vi "Initialize Sink.vi"(11 "Network Sink in":refnum<class "Network Sink.lvclass">) -> (0 "error out":errorcluster, 3 "Network Sink out":refnum<class "Network Sink.lvclass">)   [LabVIEW 2017, in "Network Sink.lvlib" / "Network Sink.lvclass"]
uses:
  <vilib>/gpm_packages/@cs/event-logger/Source/Network Sink/Network Sink/Network Sink.lvclass
  <vilib>/gpm_packages/@cs/event-logger/Source/Network Sink/Network Sink/Network Sink.lvclass/Network Sink.ctl
  <vilib>/gpm_packages/@cs/event-logger/Source/Network Sink/LogEventMessageProtocol/LogEventMessageProtocol.lvclass
  C:/Program Files/National Instruments/LabVIEW 2017/vi.lib/gpm_packages/@cs/Network-sink/Source/Network Interface/IMessagingProtocol/IMessagingProtocol.lvclass
  <vilib>/gpm_packages/@cs/Network-Sink/Source/TCP Interface/TCP Client/TCP Client.lvclass
  C:/Program Files/National Instruments/LabVIEW 2017/vi.lib/gpm_packages/@cs/Network-sink/Source/Network Interface/IConnectionFactory/IConnectionFactory.lvclass
  <vilib>/gpm_packages/@cs/event-logger/Source/Network Sink/SessionHandler/SessionHandler.lvclass
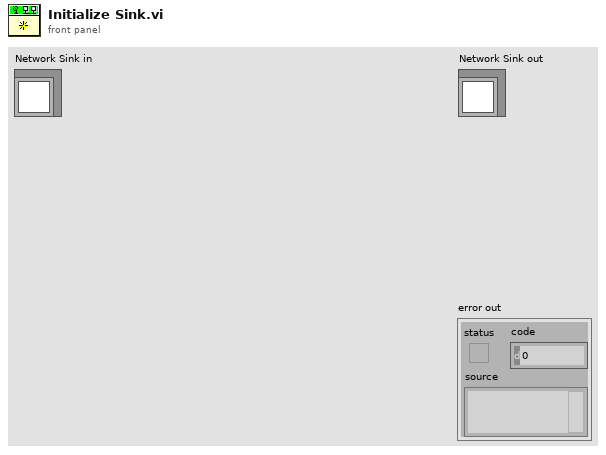
[diagram p1: front panel]
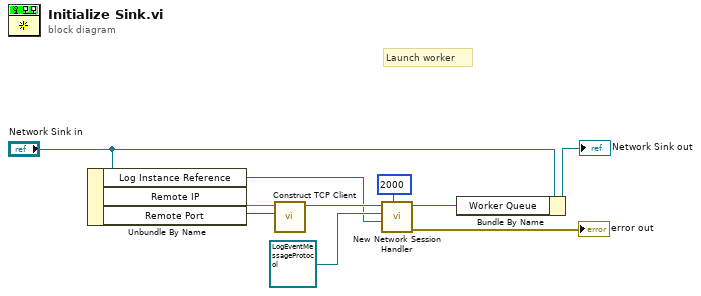
[diagram p0: block diagram]
diagram:
  # "Launch worker"
  n1 = Unbundle By Name("Network Sink in") -> ("Log Instance Reference"=w1:refnum<class "LoggerReference.lvclass">, "Remote IP"=w5:string, "Remote Port"=w4:u16)
  n2 = call <vilib>:"Construct TCP Client.vi"("Remote Port or Service Name"=w4, "Address"=w5) -> ("TCP Client out"=w2:refnum<class "TCP Client.lvclass">)  [unwired: 9 in]
  n3 = call <vilib>:"New Network Session Handler.vi"("Retry Timeout"=2000, "Log Instance Reference"=w1, "MessageProtocol"=refnum<class "LogEventMessageProtocol.lvclass"> refnum ("Network Sink.lvlib:LogEventMessageProtocol.lvclass"), "Connection Factory Type"=w2) -> ("error out"=→"error out":errorcluster, "Session Queue"=w8:refnum<queue>)  [unwired: 6 in]
  n4 = Bundle By Name(cluster="Network Sink in", "Worker Queue"=w8) -> (→"Network Sink out":refnum<class "Network Sink.lvclass">)
